vi "get_class_name.vi"(8 "error in (no error)":errorcluster, 11 "GenericPlugin in":refnum<class "GenericComponent.lvclass">) -> (0 "error out":errorcluster, 1 "class file name":string, 2 "class name":string, 3 "GenericPlugin out":refnum<class "GenericComponent.lvclass">, 4 "class file path":path)   [LabVIEW 2010, in "GenericComponent.lvclass"]
uses:
  GenericComponent.lvclass
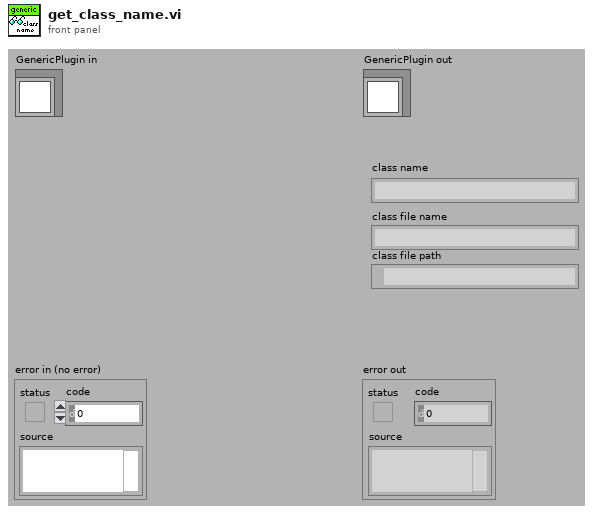
[diagram p1: front panel]
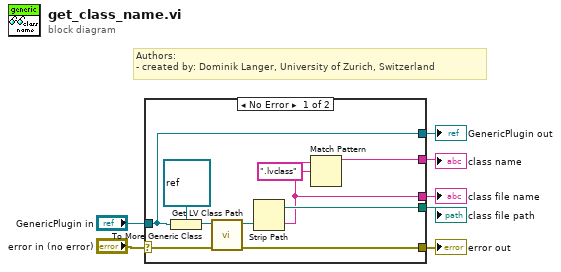
[diagram p0: block diagram]
diagram:
  # "Authors: \n- created by: Dominik Langer, University of Zurich, Switzerland"
  n1 = case shown="No Error" "error in (no error)" {
    selector: "error in (no error)" -> [w15 w19]
    tunnel: [w14 w19] -> w6
    tunnel: [w10 w18] -> w4
    tunnel: "GenericPlugin in" -> [w10 w18]
    tunnel: [w11 _] -> w3
    tunnel: [w9 _] -> w1
    tunnel: [w8 _] -> w2
    frame No Error {
      n2 = To More Generic Class(target class=refnum<class> refnum ("LabVIEW Object"), reference=w10) -> (generic class reference=w17:refnum<class>)
      n3 = call <vilib>:"Get LV Class Path.vi"("error in (no error)"=w15, "object"=w17) -> ("error out"=w14:errorcluster, "class path"=w13:path)  [unwired: 8 out]
      n4 = Strip Path(path=w13) -> (stripped path=w9:path, name=w8:string)
      n5 = Match Pattern(string=w8, regular expression=".lvclass") -> (before substring=w11:string)  [unwired: 4 out]
    }
    frame Error {
    }
  }
  "error out" <- w6
  "GenericPlugin out" <- w4
  "class name" <- w3
  "class file name" <- w2
  "class file path" <- w1
